vi "line_average.vi"(8 "error in (no error)":errorcluster, 10 "average":i32=1 min=1 step=1, 11 "AnalysisRAPS in":refnum<class "AnalysisRAPS.lvclass">) -> (0 "error out":errorcluster, 3 "AnalysisRAPS out":refnum<class "AnalysisRAPS.lvclass">)   [LabVIEW 2010, in "AnalysisRAPS.lvclass"]
uses:
  AnalysisRAPS.lvclass
  AnalysisRAPS.lvclass/AnalysisRAPS.ctl
  saving_type.ctl
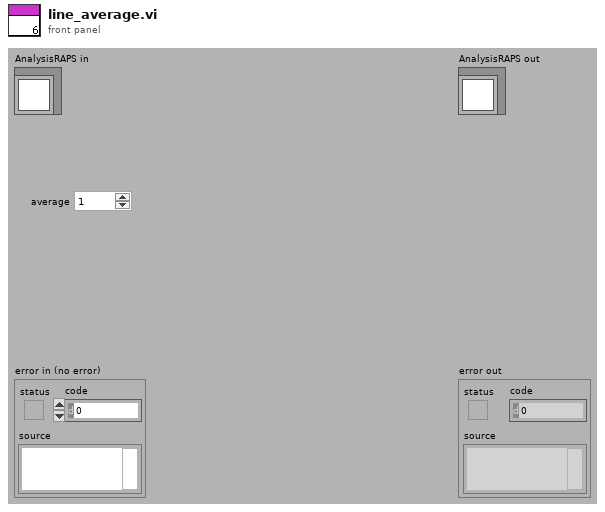
[diagram p1: front panel]
types:
  T1 = typedef "AnalysisRAPS.lvclass/saving_type.ctl" = enum16{"raw", "average"}
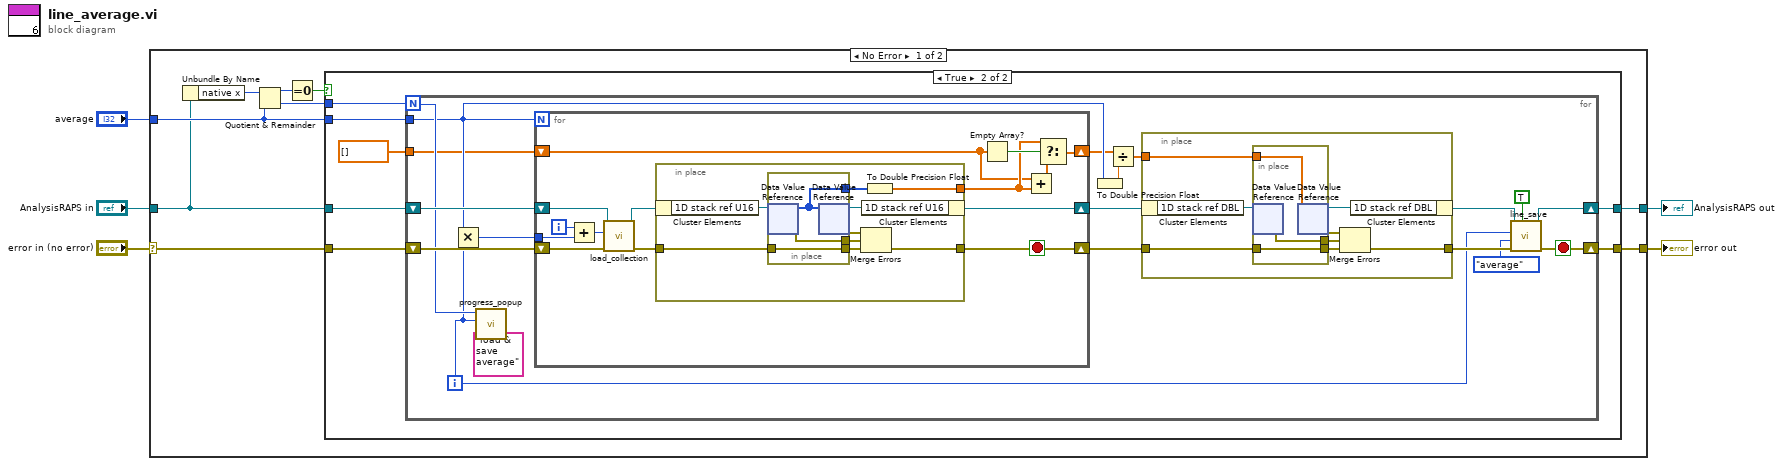
[diagram p0: block diagram]
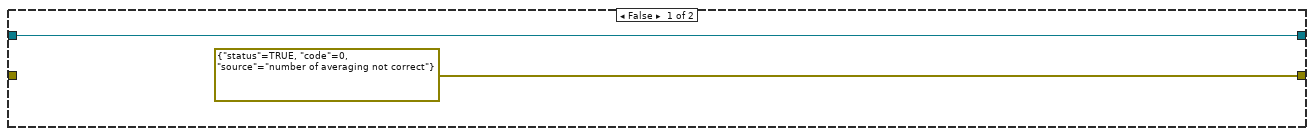
[diagram p2: hidden frame]
diagram:
  n1 = case shown="No Error" "error in (no error)" {
    selector: "error in (no error)" -> [w12 w81]
    tunnel: [w11 w81] -> w4
    tunnel: [w6 w80] -> w2
    tunnel: "AnalysisRAPS in" -> [w7 w80]
    tunnel: "average" -> [w10 _]
    frame No Error {
      n2 = Unbundle By Name(w7) -> ("native x"=w9:i32)
      n3 = Quotient & Remainder(x=w9, y=w10) -> (x-y*floor(x/y)=w14:i32, floor(x/y)=w8:i32)
      n4 = Equal To 0?(x=w14) -> (x = 0?=w13:bool)
      n5 = case shown="True" w13 {
        tunnel: [errorcluster {"status"=TRUE, "code"=0, "source"="number of averaging not correct"} ("error IO") w23] -> w11
        tunnel: w12 -> [_ w19]
        tunnel: w10 -> [_ w21]
        tunnel: w8 -> [_ w22]
        tunnel: w7 -> [w15 w20]
        tunnel: [w15 w18] -> w6
        frame False {
        }
        frame True {
          n6 = for {
            N: w22 -> [w29]
            tunnel: w21 -> [w28]
            shift-right: [w31] -> w18
            shift-left: w20 -> [w42]
            shift-right: [w32] -> w23
            shift-left: w19 -> [w33]
            tunnel: dbl[] [] -> [w24]
            i -> [w26]
            stop <- w32 stop-if-true
            n7 = Multiply(x=w28, y=w26) -> (x*y=w30:i32)
            n8 = call "progress_popup.vi"("custom text"="load & save average", "current"=w26, "total"=w29) -> ()  [unwired: 9 in]
            n9 = for {
              N: w28 -> [_]
              shift-right: [w63] -> w40
              shift-left: w42 -> [w66]
              shift-right: [w58] -> w25
              shift-left: w24 -> [w59]
              shift-right: [w57] -> w41
              shift-left: w33 -> [w67]
              tunnel: w30 -> [w56]
              i -> [w55]
              stop <- w57 stop-if-true
              n10 = Add(x=w55, y=w56) -> (x+y=w54:i32)
              n11 = call-dynamic "load_collection.vi"("error in (no error)"=w67, "index"=w54, "AnalysisRAPS in"=w66) -> ("error out"=w65:errorcluster, "AnalysisRAPS out"=w64:refnum<class "AnalysisRAPS.lvclass">)  [unwired: 7 in]
              n12 = in-place {
                in-place-border: w65 -> [w76]
                in-place-border: [w73] -> w57
                in-place-border: [w68] -> w60
                n13 = in-place-cluster #1(w64) -> ("1D stack ref U16"=w71:refnum<data-value>)
                n14 = in-place {
                  in-place-border: [w79] -> w75
                  in-place-border: [w78] -> w74
                  in-place-border: w76 -> [w78]
                  in-place-border: [w77] -> w69
                  n15 = in-place-dvr #2(w71) -> (w77:u16[], w79:errorcluster)
                  n16 = in-place-dvr #2(w77) -> (w70:refnum<data-value>, w72:errorcluster)
                }
                n17 = Merge Errors(w72, w75, w74) -> (w73:errorcluster)
                n18 = in-place-cluster #1("1D stack ref U16"=w70) -> (w63:refnum<class "AnalysisRAPS.lvclass">)
                n19 = To Double Precision Float(number=w69) -> (double precision float=w68:dbl[])
              }
              n20 = Empty Array?(array=w59) -> (empty?=w62:bool)
              n21 = Add(x=w59, y=w60) -> (x+y=w61:dbl[])
              n22 = Select(t=w60, s=w62, f=w61) -> (s? t:f=w58:dbl[])
            }
            n23 = To Double Precision Float(number=w28) -> (double precision float=w39:dbl)
            n24 = Divide(x=w25, y=w39) -> (x/y=w38:dbl[])
            n25 = in-place {
              in-place-border: w41 -> [w50]
              in-place-border: w38 -> [w45]
              in-place-border: [w43] -> w37
              n26 = in-place-cluster #3(w40) -> ("1D stack ref DBL"=w49:refnum<data-value>)
              n27 = in-place {
                in-place-border: [w53] -> w46
                in-place-border: w50 -> [w53]
                in-place-border: [w52] -> w47
                in-place-border: w45 -> [w51]
                n28 = in-place-dvr #4(w49) -> (w52:errorcluster)  [unwired: 1 out]
                n29 = in-place-dvr #4(w51) -> (w44:refnum<data-value>, w48:errorcluster)
              }
              n30 = Merge Errors(w48, w47, w46) -> (w43:errorcluster)
              n31 = in-place-cluster #3("1D stack ref DBL"=w44) -> (w35:refnum<class "AnalysisRAPS.lvclass">)
            }
            n32 = call-dynamic "line_save.vi"("double? (F)"=TRUE, "error in (no error)"=w37, "save type"=saving_type."average", "index"=w26, "AnalysisRAPS in"=w35) -> ("error out"=w32:errorcluster, "AnalysisRAPS out"=w31:refnum<class "AnalysisRAPS.lvclass">)  [unwired: 5 in]
          }
        }
      }
    }
    frame Error {
    }
  }
  "error out" <- w4
  "AnalysisRAPS out" <- w2
